vi "FreqC.Create Message Session.vi"(8 "error in":errorcluster, 10 "stop event":refnum<user-event>) -> (0 "error out":errorcluster, 2 "FreqC Message queue":refnum<queue>, 3 "FreqC Message Session out":T1)   [LabVIEW 2018]
uses:
  typedefs/FreqC.Message Session.ctl
  typedefs/FreqC.Message.ctl
  typedefs/FreqC.Message Type.ctl
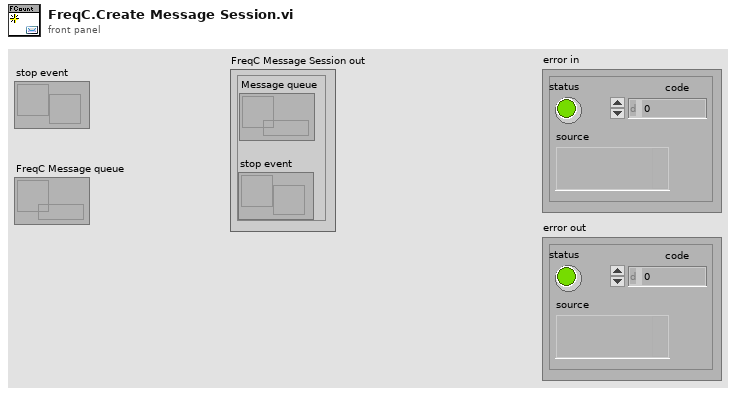
[diagram p1: front panel]
types:
  T1 = typedef "FreqC.Message Session.ctl" = cluster{"Message queue":refnum<queue>, "stop event":refnum<user-event>}
  T2 = typedef "FreqC.Message.ctl" = cluster{"Message type":T3, "data":dbl}
  T3 = typedef "FreqC.Message Type.ctl" = enum16{"meas", "set level", "set gate"}
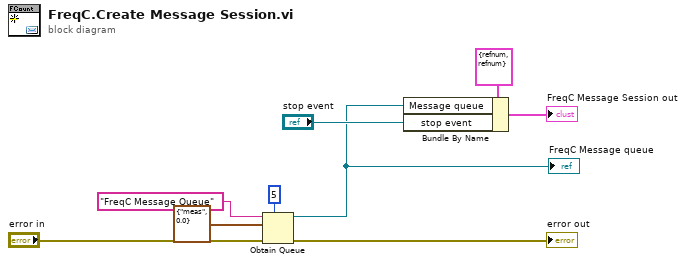
[diagram p0: block diagram]
diagram:
  n1 = Obtain Queue(max queue size (-1, unlimited)=5, name (unnamed)="FreqC Message Queue", element data type=T2 {"Message type"=enum."meas", "data"=0.0} ("FreqC.Message"), error in (no error)="error in") -> (queue out=w1:refnum<queue>, error out=→"error out":errorcluster)  [unwired: 1 in, 1 out]
  "FreqC Message queue" <- w1
  n2 = Bundle By Name(cluster=T1 {"Message queue"=refnum, "stop event"=refnum} ("FreqC.Message Session"), "Message queue"=w1, "stop event"="stop event") -> (→"FreqC Message Session out":T1)
